vi "利用组合公式求组合（化简公式）.vi"(11 "n":u32=100) -> (3 "C(n,k)":dbl)   [LabVIEW 2011]
doc: "功能：\n\n利用化简组合公式求组合。\n\n公式：\n\nC(n,k)=n!/(k!*(n-k)!\n\n根据阶乘的定义，n!可以被k!或者（n-k）的阶乘约分，因此可以选择k和n-k中较大的进行约分，极大地减少了循环次数，避免了阶乘溢出的问题。\n\n\nCSXCS_366创建"
panel:
  in  "k":u32=100
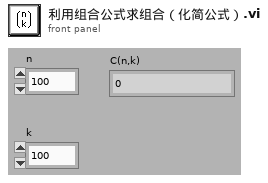
[diagram p1: front panel]
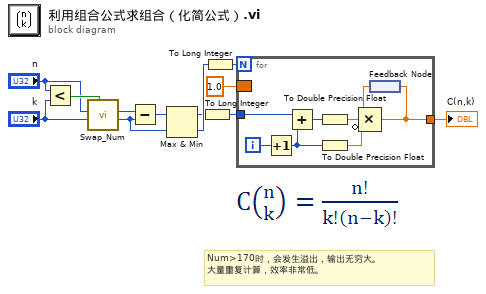
[diagram p0: block diagram]
diagram:
  # "Num>170时，会发生溢出，输出无穷大。\n大量重复计算，效率非常低。"
  n1 = Less?(x="n", y="k") -> (x < y?=w8:bool)
  n2 = call-poly "Swap_Num.vi"("Swap(T)"=w8, "b"="k", "a"="n") -> ("b"=w4:u32, "a"=w7:u32)  [unwired: 4 in]
  n3 = Subtract(x=w7, y=w4) -> (x-y=w12:u32)
  n4 = Max & Min(x=w12, y=w4) -> (max(x,y)=w10:u32, min(x,y)=w11:u32)
  n5 = To Long Integer(number=w10) -> (32bit integer=w2:i32)
  n6 = To Long Integer(number=w11) -> (32bit integer=w1:i32)
  n7 = for {
    N: w1 -> [_]
    tunnel: w2 -> [w20]
    tunnel: [w15] -> w9
    border: 1.0 ("C(n,k)") -> [_]
    i -> [w19]
    n8 = Increment(x=w19) -> (x+1=w17:i32)
    n9 = Add(x=w20, y=w17) -> (x+y=w18:i32)
    n10 = To Double Precision Float(number=w18) -> (double precision float=w14:dbl)
    n11 = To Double Precision Float(number=w17) -> (double precision float=w13:dbl)
    n12 = feedback #1() -> (w16:dbl)
    n13 = Compound Arithmetic op=MULTIPLY(w16, w14, invert w13) -> (w15:dbl)
    n14 = feedback-in #1(w15) -> ()
  }
  "C(n,k)" <- w9
